vi "VTI_Open_Queue.vi"() -> (0 "error out":errorcluster, 2 "queue out":refnum<queue>)   [LabVIEW 2019]
uses:
  S16/VTI-control.ctl
  Global/Global Variables/Queues_global.vi
panel:
  in  "error in (no error)":errorcluster
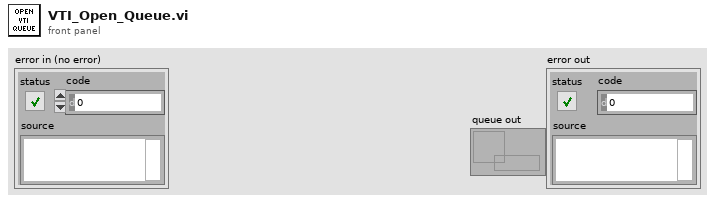
[diagram p1: front panel]
types:
  T1 = typedef "VTI-control.ctl" = cluster{"Set VTI SP":bool, "Change NV Status":bool, "Set NV Setpoint":bool, "Change Heater Status":bool, "Set Heater Setpoint":bool, "Setpoint (K)":dbl, "Rate (K/min)":dbl, "Setpoint Heater":dbl, "Setpoint NV":dbl, "Change Auto PID":bool, "Stop Sweep":bool}
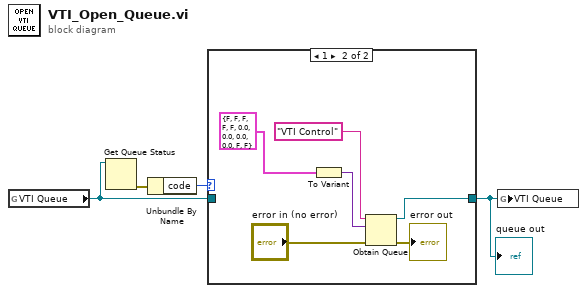
[diagram p0: block diagram]
diagram:
  n1 = global read "Queues_global.vi" "VTI Queue"() -> (w2:refnum<queue>)
  n2 = Get Queue Status(queue=w2) -> (error out=w4:errorcluster)  [unwired: 2 in, 7 out]
  n3 = Unbundle By Name(w4) -> ("code"=w3:i32)
  n4 = case shown="1" w3 {
    tunnel: [w5 w7] -> w1
    tunnel: w2 -> [w5 _]
    frame 0, Default {
    }
    frame 1 {
      n5 = To Variant(anything=T1 {"Set VTI SP"=FALSE, "Change NV Status"=FALSE, "Set NV Setpoint"=FALSE, "Change Heater Status"=FALSE, "Set Heater Setpoint"=FALSE, "Setpoint (K)"=0.0, "Rate (K/min)"=0.0, "Setpoint Heater"=0.0, "Setpoint NV"=0.0, "Change Auto PID"=FALSE, "Stop Sweep"=FALSE} ("VTI Control")) -> (Variant=w10:variant)
      n6 = Obtain Queue(name (unnamed)="VTI Control", element data type=w10, error in (no error)="error in (no error)") -> (queue out=w7:refnum<queue>, error out=→"error out":errorcluster)  [unwired: 2 in, 1 out]
    }
  }
  "queue out" <- w1
  n7 = global write "Queues_global.vi" "VTI Queue"(w1) -> ()
